vi "App - analyze RUS V6.vi"() -> ()   [LabVIEW 2015] (continued)
130814c\\5_Cooling_2nd_try\\September_2014\\091814\\14.36300K_500_2500_2.10000V_0.00000T_Sep18-2014__03-39-41_001_091814.bin", "mod time(min)"=58231179.68333333, "file format"=enum."binary", "power(V)"=2.1, "Magn Field(T) "=0.0}, {"temperature"=14.363, "temperature str"="14.36300", "file path"=path "D:/Data/Ultrasound/LSCO/LSCO22__130814c/5_Cooling_2nd_try/September_2014/091814/14.36300K_500_2500_2.10000V_0.00000T_Sep18-2014__03-41-00_001_091814.bin", "last mod"=timestamp(3493870860 s since 1904-01-01), "file name str"="D:\\Data\\Ultrasound\\LSCO\\LSCO22__130814c\\5_Cooling_2nd_try\\September_2014\\091814\\14.36300K_500_2500_2.10000V_0.00000T_Sep18-2014__03-41-00_001_091814.bin", "mod time(min)"=58231181.0, "file format"=enum."binary", "power(V)"=2.1, "Magn Field(T) "=0.0}, {"temperature"=14.36, "temperature str"="14.36000", "file path"=path "D:/Data/Ultrasound/LSCO/LSCO22__130814c/5_Cooling_2nd_try/September_2014/091814/14.36000K_500_2500_2.10000V_0.00000T_Sep18-2014__03-42-19_001_091814.bin", "last mod"=timestamp(3493870939 s since 1904-01-01), "file name str"="D:\\Data\\Ultrasound\\LSCO\\LSCO22__130814c\\5_Cooling_2nd_try\\September_2014\\091814\\14.36000K_500_2500_2.10000V_0.00000T_Sep18-2014__03-42-19_001_091814.bin", "mod time(min)"=58231182.31666667, "file format"=enum."binary", "power(V)"=2.1, "Magn Field(T) "=0.0}, {"temperature"=14.361, "temperature str"="14.36100", "file path"=path "D:/Data/Ultrasound/LSCO/LSCO22__130814c/5_Cooling_2nd_try/September_2014/091814/14.36100K_500_2500_2.10000V_0.00000T_Sep18-2014__03-43-39_001_091814.bin", "last mod"=timestamp(3493871019 s since 1904-01-01), "file name str"="D:\\Data\\Ultrasound\\LSCO\\LSCO22__130814c\\5_Cooling_2nd_try\\September_2014\\091814\\14.36100K_500_2500_2.10000V_0.00000T_Sep18-2014__03-43-39_001_091814.bin", "mod time(min)"=58231183.65, "file format"=enum."binary", "power(V)"=2.1, "Magn Field(T) "=0.0}, {"temperature"=14.361, "temperature str"="14.36100", "file path"=path "D:/Data/Ultrasound/LSCO/LSCO22__130814c/5_Cooling_2nd_try/September_2014/091814/14.36100K_500_2500_2.10000V_0.00000T_Sep18-2014__03-44-58_001_091814.bin", "last mod"=timestamp(3493871098 s since 1904-01-01), "file name str"="D:\\Data\\Ultrasound\\LSCO\\LSCO22__130814c\\5_Cooling_2nd_try\\September_2014\\091814\\14.36100K_500_2500_2.10000V_0.00000T_Sep18-2014__03-44-58_001_091814.bin", "mod time(min)"=58231184.96666667, "file format"=enum."binary", "power(V)"=2.1, "Magn Field(T) "=0.0}, {"temperature"=14.357, "temperature str"="14.35700", "file path"=path "D:/Data/Ultrasound/LSCO/LSCO22__130814c/5_Cooling_2nd_try/September_2014/091814/14.35700K_500_2500_2.10000V_0.00000T_Sep18-2014__03-46-18_001_091814.bin", "last mod"=timestamp(3493871178 s since 1904-01-01), "file name str"="D:\\Data\\Ultrasound\\LSCO\\LSCO22__130814c\\5_Cooling_2nd_try\\September_2014\\091814\\14.35700K_500_2500_2.10000V_0.00000T_Sep18-2014__03-46-18_001_091814.bin", "mod time(min)"=58231186.3, "file format"=enum."binary", "power(V)"=2.1, "Magn Field(T) "=0.0}, {"temperature"=14.357, "temperature str"="14.35700", "file path"=path "D:/Data/Ultrasound/LSCO/LSCO22__130814c/5_Cooling_2nd_try/September_2014/091814/14.35700K_500_2500_2.10000V_0.00000T_Sep18-2014__03-47-37_001_091814.bin", "last mod"=timestamp(3493871257 s since 1904-01-01), "file name str"="D:\\Data\\Ultrasound\\LSCO\\LSCO22__130814c\\5_Cooling_2nd_try\\September_2014\\091814\\14.35700K_500_2500_2.10000V_0.00000T_Sep18-2014__03-47-37_001_091814.bin", "mod time(min)"=58231187.61666667, "file format"=enum."binary", "power(V)"=2.1, "Magn Field(T) "=0.0}, {"temperature"=14.355, "temperature str"="14.35500", "file path"=path "D:/Data/Ultrasound/LSCO/LSCO22__130814c/5_Cooling_2nd_try/September_2014/091814/14.35500K_500_2500_2.10000V_0.00000T_Sep18-2014__03-48-56_001_091814.bin", "last mod"=timestamp(3493871336 s since 1904-01-01), "file name str"="D:\\Data\\Ultrasound\\LSCO\\LSCO22__130814c\\5_Cooling_2nd_try\\September_2014\\091814\\14.35500K_500_2500_2.10000V_0.00000T_Sep18-2014__03-48-56_001_091814.bin", "mod time(min)"=58231188.93333333, "file format"=enum."binary", "power(V)"=2.1, "Magn Field(T) "=0.0}, {"temperature"=14.354, "temperature str"="14.35400", "file path"=path "D:/Data/Ultrasound/LSCO/LSCO22__130814c/5_Cooling_2nd_try/September_2014/091814/14.35400K_500_2500_2.10000V_0.00000T_Sep18-2014__03-50-16_001_091814.bin", "last mod"=timestamp(3493871416 s since 1904-01-01), "file name str"="D:\\Data\\Ultrasound\\LSCO\\LSCO22__130814c\\5_Cooling_2nd_try\\September_2014\\091814\\14.35400K_500_2500_2.10000V_0.00000T_Sep18-2014__03-50-16_001_091814.bin", "mod time(min)"=58231190.266666666, "file format"=enum."binary", "power(V)"=2.1, "Magn Field(T) "=0.0}, {"temperature"=14.354, "temperature str"="14.35400", "file path"=path "D:/Data/Ultrasound/LSCO/LSCO22__130814c/5_Cooling_2nd_try/September_2014/091814/14.35400K_500_2500_2.10000V_0.00000T_Sep18-2014__03-51-35_001_091814.bin", "last mod"=timestamp(3493871495 s since 1904-01-01), "file name str"="D:\\Data\\Ultrasound\\LSCO\\LSCO22__130814c\\5_Cooling_2nd_try\\September_2014\\091814\\14.35400K_500_2500_2.10000V_0.00000T_Sep18-2014__03-51-35_001_091814.bin", "mod time(min)"=58231191.583333336, "file format"=enum."binary", "power(V)"=2.1, "Magn Field(T) "=0.0}, {"temperature"=14.352, "temperature str"="14.35200", "file path"=path "D:/Data/Ultrasound/LSCO/LSCO22__130814c/5_Cooling_2nd_try/September_2014/091814/14.35200K_500_2500_2.10000V_0.00000T_Sep18-2014__03-52-54_001_091814.bin", "last mod"=timestamp(3493871574 s since 1904-01-01), "file name str"="D:\\Data\\Ultrasound\\LSCO\\LSCO22__130814c\\5_Cooling_2nd_try\\September_2014\\091814\\14.35200K_500_2500_2.10000V_0.00000T_Sep18-2014__03-52-54_001_091814.bin", "mod time(min)"=58231192.9, "file format"=enum."binary", "power(V)"=2.1, "Magn Field(T) "=0.0}, {"temperature"=14.349, "temperature str"="14.34900", "file path"=path "D:/Data/Ultrasound/LSCO/LSCO22__130814c/5_Cooling_2nd_try/September_2014/091814/14.34900K_500_2500_2.10000V_0.00000T_Sep18-2014__03-54-14_001_091814.bin", "last mod"=timestamp(3493871654 s since 1904-01-01), "file name str"="D:\\Data\\Ultrasound\\LSCO\\LSCO22__130814c\\5_Cooling_2nd_try\\September_2014\\091814\\14.34900K_500_2500_2.10000V_0.00000T_Sep18-2014__03-54-14_001_091814.bin", "mod time(min)"=58231194.233333334, "file format"=enum."binary", "power(V)"=2.1, "Magn Field(T) "=0.0}, {"temperature"=14.353, "temperature str"="14.35300", "file path"=path "D:/Data/Ultrasound/LSCO/LSCO22__130814c/5_Cooling_2nd_try/September_2014/091814/14.35300K_500_2500_2.10000V_0.00000T_Sep18-2014__03-55-33_001_091814.bin", "last mod"=timestamp(3493871733 s since 1904-01-01), "file name str"="D:\\Data\\Ultrasound\\LSCO\\LSCO22__130814c\\5_Cooling_2nd_try\\September_2014\\091814\\14.35300K_500_2500_2.10000V_0.00000T_Sep18-2014__03-55-33_001_091814.bin", "mod time(min)"=58231195.55, "file format"=enum."binary", "power(V)"=2.1, "Magn Field(T) "=0.0}, {"temperature"=14.35, "temperature str"="14.35000", "file path"=path "D:/Data/Ultrasound/LSCO/LSCO22__130814c/5_Cooling_2nd_try/September_2014/091814/14.35000K_500_2500_2.10000V_0.00000T_Sep18-2014__03-56-53_001_091814.bin", "last mod"=timestamp(3493871813 s since 1904-01-01), "file name str"="D:\\Data\\Ultrasound\\LSCO\\LSCO22__130814c\\5_Cooling_2nd_try\\September_2014\\091814\\14.35000K_500_2500_2.10000V_0.00000T_Sep18-2014__03-56-53_001_091814.bin", "mod time(min)"=58231196.88333333, "file format"=enum."binary", "power(V)"=2.1, "Magn Field(T) "=0.0}, {"temperature"=14.351, "temperature str"="14.35100", "file path"=path "D:/Data/Ultrasound/LSCO/LSCO22__130814c/5_Cooling_2nd_try/September_2014/091814/14.35100K_500_2500_2.10000V_0.00000T_Sep18-2014__03-58-12_001_091814.bin", "last mod"=timestamp(3493871892 s since 1904-01-01), "file name str"="D:\\Data\\Ultrasound\\LSCO\\LSCO22__130814c\\5_Cooling_2nd_try\\September_2014\\091814\\14.35100K_500_2500_2.10000V_0.00000T_Sep18-2014__03-58-12_001_091814.bin", "mod time(min)"=58231198.2, "file format"=enum."binary", "power(V)"=2.1, "Magn Field(T) "=0.0}, {"temperature"=14.351, "temperature str"="14.35100", "file path"=path "D:/Data/Ultrasound/LSCO/LSCO22__130814c/5_Cooling_2nd_try/September_2014/091814/14.35100K_500_2500_2.10000V_0.00000T_Sep18-2014__03-59-31_001_091814.bin", "last mod"=timestamp(3493871971 s since 1904-01-01), "file name str"="D:\\Data\\Ultrasound\\LSCO\\LSCO22__130814c\\5_Cooling_2nd_try\\September_2014\\091814\\14.35100K_500_2500_2.10000V_0.00000T_Sep18-2014__03-59-31_001_091814.bin", "mod time(min)"=58231199.516666666, "file format"=enum."binary", "power(V)"=2.1, "Magn Field(T) "=0.0}, {"temperature"=14.353, "temperature str"="14.35300", "file path"=path "D:/Data/Ultrasound/LSCO/LSCO22__130814c/5_Cooling_2nd_try/September_2014/091814/14.35300K_500_2500_2.10000V_0.00000T_Sep18-2014__04-00-51_001_091814.bin", "last mod"=timestamp(3493872051 s since 1904-01-01), "file name str"="D:\\Data\\Ultrasound\\LSCO\\LSCO22__130814c\\5_Cooling_2nd_try\\September_2014\\091814\\14.35300K_500_2500_2.10000V_0.00000T_Sep18-2014__04-00-51_001_091814.bin", "mod time(min)"=58231200.85, "file format"=enum."binary", "power(V)"=2.1, "Magn Field(T) "=0.0}, {"temperature"=14.352, "temperature str"="14.35200", "file path"=path "D:/Data/Ultrasound/LSCO/LSCO22__130814c/5_Cooling_2nd_try/September_2014/091814/14.35200K_500_2500_2.10000V_0.00000T_Sep18-2014__04-02-10_001_091814.bin", "last mod"=timestamp(3493872130 s since 1904-01-01), "file name str"="D:\\Data\\Ultrasound\\LSCO\\LSCO22__130814c\\5_Cooling_2nd_try\\September_2014\\091814\\14.35200K_500_2500_2.10000V_0.00000T_Sep18-2014__04-02-10_001_091814.bin", "mod time(min)"=58231202.166666664, "file format"=enum."binary", "power(V)"=2.1, "Magn Field(T) "=0.0}, {"temperature"=14.354, "temperature str"="14.35400", "file path"=path "D:/Data/Ultrasound/LSCO/LSCO22__130814c/5_Cooling_2nd_try/September_2014/091814/14.35400K_500_2500_2.10000V_0.00000T_Sep18-2014__04-03-30_001_091814.bin", "last mod"=timestamp(3493872210 s since 1904-01-01), "file name str"="D:\\Data\\Ultrasound\\LSCO\\LSCO22__130814c\\5_Cooling_2nd_try\\September_2014\\091814\\14.35400K_500_2500_2.10000V_0.00000T_Sep18-2014__04-03-30_001_091814.bin", "mod time(min)"=58231203.5, "file format"=enum."binary", "power(V)"=2.1, "Magn Field(T) "=0.0}, {"temperature"=14.354, "temperature str"="14.35400", "file path"=path "D:/Data/Ultrasound/LSCO/LSCO22__130814c/5_Cooling_2nd_try/September_2014/091814/14.35400K_500_2500_2.10000V_0.00000T_Sep18-2014__04-04-49_001_091814.bin", "last mod"=timestamp(3493872289 s since 1904-01-01), "file name str"="D:\\Data\\Ultrasound\\LSCO\\LSCO22__130814c\\5_Cooling_2nd_try\\September_2014\\091814\\14.35400K_500_2500_2.10000V_0.00000T_Sep18-2014__04-04-49_001_091814.bin", "mod time(min)"=58231204.81666667, "file format"=enum."binary", "power(V)"=2.1, "Magn Field(T) "=0.0}, {"temperature"=14.358, "temperature str"="14.35800", "file path"=path "D:/Data/Ultrasound/LSCO/LSCO22__130814c/5_Cooling_2nd_try/September_2014/091814/14.35800K_500_2500_2.10000V_0.00000T_Sep18-2014__04-06-08_001_091814.bin", "last mod"=timestamp(3493872368 s since 1904-01-01), "file name str"="D:\\Data\\Ultrasound\\LSCO\\LSCO22__130814c\\5_Cooling_2nd_try\\September_2014\\091814\\14.35800K_500_2500_2.10000V_0.00000T_Sep18-2014__04-06-08_001_091814.bin", "mod time(min)"=58231206.13333333, "file format"=enum."binary", "power(V)"=2.1, "Magn Field(T) "=0.0}, {"temperature"=14.357, "temperature str"="14.35700", "file path"=path "D:/Data/Ultrasound/LSCO/LSCO22__130814c/5_Cooling_2nd_try/September_2014/091814/14.35700K_500_2500_2.10000V_0.00000T_Sep18-2014__04-07-28_001_091814.bin", "last mod"=timestamp(3493872448 s since 1904-01-01), "file name str"="D:\\Data\\Ultrasound\\LSCO\\LSCO22__130814c\\5_Cooling_2nd_try\\September_2014\\091814\\14.35700K_500_2500_2.10000V_0.00000T_Sep18-2014__04-07-28_001_091814.bin", "mod time(min)"=58231207.46666667, "file format"=enum."binary", "power(V)"=2.1, "Magn Field(T) "=0.0}, {"temperature"=14.356, "temperature str"="14.35600", "file path"=path "D:/Data/Ultrasound/LSCO/LSCO22__130814c/5_Cooling_2nd_try/September_2014/091814/14.35600K_500_2500_2.10000V_0.00000T_Sep18-2014__04-08-47_001_091814.bin", "last mod"=timestamp(3493872527 s since 1904-01-01), "file name str"="D:\\Data\\Ultrasound\\LSCO\\LSCO22__130814c\\5_Cooling_2nd_try\\September_2014\\091814\\14.35600K_500_2500_2.10000V_0.00000T_Sep18-2014__04-08-47_001_091814.bin", "mod time(min)"=58231208.78333333, "file format"=enum."binary", "power(V)"=2.1, "Magn Field(T) "=0.0}, {"temperature"=14.356, "temperature str"="14.35600", "file path"=path "D:/Data/Ultrasound/LSCO/LSCO22__130814c/5_Cooling_2nd_try/September_2014/091814/14.35600K_500_2500_2.10000V_0.00000T_Sep18-2014__04-10-06_001_091814.bin", "last mod"=timestamp(3493872606 s since 1904-01-01), "file name str"="D:\\Data\\Ultrasound\\LSCO\\LSCO22__130814c\\5_Cooling_2nd_try\\September_2014\\091814\\14.35600K_500_2500_2.10000V_0.00000T_Sep18-2014__04-10-06_001_091814.bin", "mod time(min)"=58231210.1, "file format"=enum."binary", "power(V)"=2.1, "Magn Field(T) "=0.0}, {"temperature"=14.354, "temperature str"="14.35400", "file path"=path "D:/Data/Ultrasound/LSCO/LSCO22__130814c/5_Cooling_2nd_try/September_2014/091814/14.35400K_500_2500_2.10000V_0.00000T_Sep18-2014__04-11-26_001_091814.bin", "last mod"=timestamp(3493872686 s since 1904-01-01), "file name str"="D:\\Data\\Ultrasound\\LSCO\\LSCO22__130814c\\5_Cooling_2nd_try\\September_2014\\091814\\14.35400K_500_2500_2.10000V_0.00000T_Sep18-2014__04-11-26_001_091814.bin", "mod time(min)"=58231211.43333333, "file format"=enum."binary", "power(V)"=2.1, "Magn Field(T) "=0.0}, {"temperature"=14.35, "temperature str"="14.35000", "file path"=path "D:/Data/Ultrasound/LSCO/LSCO22__130814c/5_Cooling_2nd_try/September_2014/091814/14.35000K_500_2500_2.10000V_0.00000T_Sep18-2014__04-12-45_001_091814.bin", "last mod"=timestamp(3493872765 s since 1904-01-01), "file name str"="D:\\Data\\Ultrasound\\LSCO\\LSCO22__130814c\\5_Cooling_2nd_try\\September_2014\\091814\\14.35000K_500_2500_2.10000V_0.00000T_Sep18-2014__04-12-45_001_091814.bin", "mod time(min)"=58231212.75, "file format"=enum."binary", "power(V)"=2.1, "Magn Field(T) "=0.0}, {"temperature"=14.352, "temperature str"="14.35200", "file path"=path "D:/Data/Ultrasound/LSCO/LSCO22__130814c/5_Cooling_2nd_try/September_2014/091814/14.35200K_500_2500_2.10000V_0.00000T_Sep18-2014__04-14-05_001_091814.bin", "last mod"=timestamp(3493872845 s since 1904-01-01), "file name str"="D:\\Data\\Ultrasound\\LSCO\\LSCO22__130814c\\5_Cooling_2nd_try\\September_2014\\091814\\14.35200K_500_2500_2.10000V_0.00000T_Sep18-2014__04-14-05_001_091814.bin", "mod time(min)"=58231214.083333336, "file format"=enum."binary", "power(V)"=2.1, "Magn Field(T) "=0.0}, {"temperature"=14.354, "temperature str"="14.35400", "file path"=path "D:/Data/Ultrasound/LSCO/LSCO22__130814c/5_Cooling_2nd_try/September_2014/091814/14.35400K_500_2500_2.10000V_0.00000T_Sep18-2014__04-15-24_001_091814.bin", "last mod"=timestamp(3493872924 s since 1904-01-01), "file name str"="D:\\Data\\Ultrasound\\LSCO\\LSCO22__130814c\\5_Cooling_2nd_try\\September_2014\\091814\\14.35400K_500_2500_2.10000V_0.00000T_Sep18-2014__04-15-24_001_091814.bin", "mod time(min)"=58231215.4, "file format"=enum."binary", "power(V)"=2.1, "Magn Field(T) "=0.0}, {"temperature"=14.349, "temperature str"="14.34900", "file path"=path "D:/Data/Ultrasound/LSCO/LSCO22__130814c/5_Cooling_2nd_try/September_2014/091814/14.34900K_500_2500_2.10000V_0.00000T_Sep18-2014__04-16-43_001_091814.bin", "last mod"=timestamp(3493873003 s since 1904-01-01), "file name str"="D:\\Data\\Ultrasound\\LSCO\\LSCO22__130814c\\5_Cooling_2nd_try\\September_2014\\091814\\14.34900K_500_2500_2.10000V_0.00000T_Sep18-2014__04-16-43_001_091814.bin", "mod time(min)"=58231216.71666667, "file format"=enum."binary", "power(V)"=2.1, "Magn Field(T) "=0.0}, {"temperature"=14.349, "temperature str"="14.34900", "file path"=path "D:/Data/Ultrasound/LSCO/LSCO22__130814c/5_Cooling_2nd_try/September_2014/091814/14.34900K_500_2500_2.10000V_0.00000T_Sep18-2014__04-18-03_001_091814.bin", "last mod"=timestamp(3493873083 s since 1904-01-01), "file name str"="D:\\Data\\Ultrasound\\LSCO\\LSCO22__130814c\\5_Cooling_2nd_try\\September_2014\\091814\\14.34900K_500_2500_2.10000V_0.00000T_Sep18-2014__04-18-03_001_091814.bin", "mod time(min)"=58231218.05, "file format"=enum."binary", "power(V)"=2.1, "Magn Field(T) "=0.0}, {"temperature"=14.346, "temperature str"="14.34600", "file path"=path "D:/Data/Ultrasound/LSCO/LSCO22__130814c/5_Cooling_2nd_try/September_2014/091814/14.34600K_500_2500_2.10000V_0.00000T_Sep18-2014__04-19-22_001_091814.bin", "last mod"=timestamp(3493873162 s since 1904-01-01), "file name str"="D:\\Data\\Ultrasound\\LSCO\\LSCO22__130814c\\5_Cooling_2nd_try\\September_2014\\091814\\14.34600K_500_2500_2.10000V_0.00000T_Sep18-2014__04-19-22_001_091814.bin", "mod time(min)"=58231219.36666667, "file format"=enum."binary", "power(V)"=2.1, "Magn Field(T) "=0.0}, {"temperature"=14.344, "temperature str"="14.34400", "file path"=path "D:/Data/Ultrasound/LSCO/LSCO22__130814c/5_Cooling_2nd_try/September_2014/091814/14.34400K_500_2500_2.10000V_0.00000T_Sep18-2014__04-20-42_001_091814.bin", "last mod"=timestamp(3493873242 s since 1904-01-01), "file name str"="D:\\Data\\Ultrasound\\LSCO\\LSCO22__130814c\\5_Cooling_2nd_try\\September_2014\\091814\\14.34400K_500_2500_2.10000V_0.00000T_Sep18-2014__04-20-42_001_091814.bin", "mod time(min)"=58231220.7, "file format"=enum."binary", "power(V)"=2.1, "Magn Field(T) "=0.0}, {"temperature"=14.346, "temperature str"="14.34600", "file path"=path "D:/Data/Ultrasound/LSCO/LSCO22__130814c/5_Cooling_2nd_try/September_2014/091814/14.34600K_500_2500_2.10000V_0.00000T_Sep18-2014__04-22-01_001_091814.bin", "last mod"=timestamp(3493873321 s since 1904-01-01), "file name str"="D:\\Data\\Ultrasound\\LSCO\\LSCO22__130814c\\5_Cooling_2nd_try\\September_2014\\091814\\14.34600K_500_2500_2.10000V_0.00000T_Sep18-2014__04-22-01_001_091814.bin", "mod time(min)"=58231222.016666666, "file format"=enum."binary", "power(V)"=2.1, "Magn Field(T) "=0.0}, {"temperature"=14.346, "temperature str"="14.34600", "file path"=path "D:/Data/Ultrasound/LSCO/LSCO22__130814c/5_Cooling_2nd_try/September_2014/091814/14.34600K_500_2500_2.10000V_0.00000T_Sep18-2014__04-23-20_001_091814.bin", "last mod"=timestamp(3493873400 s since 1904-01-01), "file name str"="D:\\Data\\Ultrasound\\LSCO\\LSCO22__130814c\\5_Cooling_2nd_try\\September_2014\\091814\\14.34600K_500_2500_2.10000V_0.00000T_Sep18-2014__04-23-20_001_091814.bin", "mod time(min)"=58231223.333333336, "file format"=enum."binary", "power(V)"=2.1, "Magn Field(T) "=0.0}, {"temperature"=14.348, "temperature str"="14.34800", "file path"=path "D:/Data/Ultrasound/LSCO/LSCO22__130814c/5_Cooling_2nd_try/September_2014/091814/14.34800K_500_2500_2.10000V_0.00000T_Sep18-2014__04-24-40_001_091814.bin", "last mod"=timestamp(3493873480 s since 1904-01-01), "file name str"="D:\\Data\\Ultrasound\\LSCO\\LSCO22__130814c\\5_Cooling_2nd_try\\September_2014\\091814\\14.34800K_500_2500_2.10000V_0.00000T_Sep18-2014__04-24-40_001_091814.bin", "mod time(min)"=58231224.666666664, "file format"=enum."binary", "power(V)"=2.1, "Magn Field(T) "=0.0}, {"temperature"=14.353, "temperature str"="14.35300", "file path"=path "D:/Data/Ultrasound/LSCO/LSCO22__130814c/5_Cooling_2nd_try/September_2014/091814/14.35300K_500_2500_2.10000V_0.00000T_Sep18-2014__04-25-59_001_091814.bin", "last mod"=timestamp(3493873559 s since 1904-01-01), "file name str"="D:\\Data\\Ultrasound\\LSCO\\LSCO22__130814c\\5_Cooling_2nd_try\\September_2014\\091814\\14.35300K_500_2500_2.10000V_0.00000T_Sep18-2014__04-25-59_001_091814.bin", "mod time(min)"=58231225.983333334, "file format"=enum."binary", "power(V)"=2.1, "Magn Field(T) "=0.0}, {"temperature"=14.355, "temperature str"="14.35500", "file path"=path "D:/Data/Ultrasound/LSCO/LSCO22__130814c/5_Cooling_2nd_try/September_2014/091814/14.35500K_500_2500_2.10000V_0.00000T_Sep18-2014__04-27-18_001_091814.bin", "last mod"=timestamp(3493873638 s since 1904-01-01), "file name str"="D:\\Data\\Ultrasound\\LSCO\\LSCO22__130814c\\5_Cooling_2nd_try\\September_2014\\091814\\14.35500K_500_2500_2.10000V_0.00000T_Sep18-2014__04-27-18_001_091814.bin", "mod time(min)"=58231227.3, "file format"=enum."binary", "power(V)"=2.1, "Magn Field(T) "=0.0}, {"temperature"=14.349, "temperature str"="14.34900", "file path"=path "D:/Data/Ultrasound/LSCO/LSCO22__130814c/5_Cooling_2nd_try/September_2014/091814/14.34900K_500_2500_2.10000V_0.00000T_Sep18-2014__04-28-38_001_091814.bin", "last mod"=timestamp(3493873718 s since 1904-01-01), "file name str"="D:\\Data\\Ultrasound\\LSCO\\LSCO22__130814c\\5_Cooling_2nd_try\\September_2014\\091814\\14.34900K_500_2500_2.10000V_0.00000T_Sep18-2014__04-28-38_001_091814.bin", "mod time(min)"=58231228.63333333, "file format"=enum."binary", "power(V)"=2.1, "Magn Field(T) "=0.0}, {"temperature"=14.351, "temperature str"="14.35100", "file path"=path "D:/Data/Ultrasound/LSCO/LSCO22__130814c/5_Cooling_2nd_try/September_2014/091814/14.35100K_500_2500_2.10000V_0.00000T_Sep18-2014__04-29-57_001_091814.bin", "last mod"=timestamp(3493873797 s since 1904-01-01), "file name str"="D:\\Data\\Ultrasound\\LSCO\\LSCO22__130814c\\5_Cooling_2nd_try\\September_2014\\091814\\14.35100K_500_2500_2.10000V_0.00000T_Sep18-2014__04-29-57_001_091814.bin", "mod time(min)"=58231229.95, "file format"=enum."binary", "power(V)"=2.1, "Magn Field(T) "=0.0}, {"temperature"=14.35, "temperature str"="14.35000", "file path"=path "D:/Data/Ultrasound/LSCO/LSCO22__130814c/5_Cooling_2nd_try/September_2014/091814/14.35000K_500_2500_2.10000V_0.00000T_Sep18-2014__04-31-17_001_091814.bin", "last mod"=timestamp(3493873877 s since 1904-01-01), "file name str"="D:\\Data\\Ultrasound\\LSCO\\LSCO22__130814c\\5_Cooling_2nd_try\\September_2014\\091814\\14.35000K_500_2500_2.10000V_0.00000T_Sep18-2014__04-31-17_001_091814.bin", "mod time(min)"=58231231.28333333, "file format"=enum."binary", "power(V)"=2.1, "Magn Field(T) "=0.0}, {"temperature"=14.347, "temperature str"="14.34700", "file path"=path "D:/Data/Ultrasound/LSCO/LSCO22__130814c/5_Cooling_2nd_try/September_2014/091814/14.34700K_500_2500_2.10000V_0.00000T_Sep18-2014__04-32-36_001_091814.bin", "last mod"=timestamp(3493873956 s since 1904-01-01), "file name str"="D:\\Data\\Ultrasound\\LSCO\\LSCO22__130814c\\5_Cooling_2nd_try\\September_2014\\091814\\14.34700K_500_2500_2.10000V_0.00000T_Sep18-2014__04-32-36_001_091814.bin", "mod time(min)"=58231232.6, "file format"=enum."binary", "power(V)"=2.1, "Magn Field(T) "=0.0}, {"temperature"=14.35, "temperature str"="14.35000", "file path"=path "D:/Data/Ultrasound/LSCO/LSCO22__130814c/5_Cooling_2nd_try/September_2014/091814/14.35000K_500_2500_2.10000V_0.00000T_Sep18-2014__04-33-55_001_091814.bin", "last mod"=timestamp(3493874035 s since 1904-01-01), "file name str"="D:\\Data\\Ultrasound\\LSCO\\LSCO22__130814c\\5_Cooling_2nd_try\\September_2014\\091814\\14.35000K_500_2500_2.10000V_0.00000T_Sep18-2014__04-33-55_001_091814.bin", "mod time(min)"=58231233.916666664, "file format"=enum."binary", "power(V)"=2.1, "Magn Field(T) "=0.0}, {"temperature"=14.349, "temperature str"="14.34900", "file path"=path "D:/Data/Ultrasound/LSCO/LSCO22__130814c/5_Cooling_2nd_try/September_2014/091814/14.34900K_500_2500_2.10000V_0.00000T_Sep18-2014__04-35-15_001_091814.bin", "last mod"=timestamp(3493874115 s since 1904-01-01), "file name str"="D:\\Data\\Ultrasound\\LSCO\\LSCO22__130814c\\5_Cooling_2nd_try\\September_2014\\091814\\14.34900K_500_2500_2.10000V_0.00000T_Sep18-2014__04-35-15_001_091814.bin", "mod time(min)"=58231235.25, "file format"=enum."binary", "power(V)"=2.1, "Magn Field(T) "=0.0}, {"temperature"=14.35, "temperature str"="14.35000", "file path"=path "D:/Data/Ultrasound/LSCO/LSCO22__130814c/5_Cooling_2nd_try/September_2014/091814/14.35000K_500_2500_2.10000V_0.00000T_Sep18-2014__04-36-34_001_091814.bin", "last mod"=timestamp(3493874194 s since 1904-01-01), "file name str"="D:\\Data\\Ultrasound\\LSCO\\LSCO22__130814c\\5_Cooling_2nd_try\\September_2014\\091814\\14.35000K_500_2500_2.10000V_0.00000T_Sep18-2014__04-36-34_001_091814.bin", "mod time(min)"=58231236.56666667, "file format"=enum."binary", "power(V)"=2.1, "Magn Field(T) "=0.0}, {"temperature"=14.351, "temperature str"="14.35100", "file path"=path "D:/Data/Ultrasound/LSCO/LSCO22__130814c/5_Cooling_2nd_try/September_2014/091814/14.35100K_500_2500_2.10000V_0.00000T_Sep18-2014__04-37-53_001_091814.bin", "last mod"=timestamp(3493874273 s since 1904-01-01), "file name str"="D:\\Data\\Ultrasound\\LSCO\\LSCO22__130814c\\5_Cooling_2nd_try\\September_2014\\091814\\14.35100K_500_2500_2.10000V_0.00000T_Sep18-2014__04-37-53_001_091814.bin", "mod time(min)"=58231237.88333333, "file format"=enum."binary", "power(V)"=2.1, "Magn Field(T) "=0.0}, {"temperature"=14.351, "temperature str"="14.35100", "file path"=path "D:/Data/Ultrasound/LSCO/LSCO22__130814c/5_Cooling_2nd_try/September_2014/091814/14.35100K_500_2500_2.10000V_0.00000T_Sep18-2014__04-39-13_001_091814.bin", "last mod"=timestamp(3493874353 s since 1904-01-01), "file name str"="D:\\Data\\Ultrasound\\LSCO\\LSCO22__130814c\\5_Cooling_2nd_try\\September_2014\\091814\\14.35100K_500_2500_2.10000V_0.00000T_Sep18-2014__04-39-13_001_091814.bin", "mod time(min)"=58231239.21666667, "file format"=enum."binary", "power(V)"=2.1, "Magn Field(T) "=0.0}, {"temperature"=14.352, "temperature str"="14.35200", "file path"=path "D:/Data/Ultrasound/LSCO/LSCO22__130814c/5_Cooling_2nd_try/September_2014/091814/14.35200K_500_2500_2.10000V_0.00000T_Sep18-2014__04-40-32_001_091814.bin", "last mod"=timestamp(3493874432 s since 1904-01-01), "file name str"="D:\\Data\\Ultrasound\\LSCO\\LSCO22__130814c\\5_Cooling_2nd_try\\September_2014\\091814\\14.35200K_500_2500_2.10000V_0.00000T_Sep18-2014__04-40-32_001_091814.bin", "mod time(min)"=58231240.53333333, "file format"=enum."binary", "power(V)"=2.1, "Magn Field(T) "=0.0}, {"temperature"=14.351, "temperature str"="14.35100", "file path"=path "D:/Data/Ultrasound/LSCO/LSCO22__130814c/5_Cooling_2nd_try/September_2014/091814/14.35100K_500_2500_2.10000V_0.00000T_Sep18-2014__04-41-52_001_091814.bin", "last mod"=timestamp(3493874512 s since 1904-01-01), "file name str"="D:\\Data\\Ultrasound\\LSCO\\LSCO22__130814c\\5_Cooling_2nd_try\\September_2014\\091814\\14.35100K_500_2500_2.10000V_0.00000T_Sep18-2014__04-41-52_001_091814.bin", "mod time(min)"=58231241.86666667, "file format"=enum."binary", "power(V)"=2.1, "Magn Field(T) "=0.0}, {"temperature"=14.35, "temperature str"="14.35000", "file path"=path "D:/Data/Ultrasound/LSCO/LSCO22__130814c/5_Cooling_2nd_try/September_2014/091814/14.35000K_500_2500_2.10000V_0.00000T_Sep18-2014__04-43-11_001_091814.bin", "last mod"=timestamp(3493874591 s since 1904-01-01), "file name str"="D:\\Data\\Ultrasound\\LSCO\\LSCO22__130814c\\5_Cooling_2nd_try\\September_2014\\091814\\14.35000K_500_2500_2.10000V_0.00000T_Sep18-2014__04-43-11_001_091814.bin", "mod time(min)"=58231243.18333333, "file format"=enum."binary", "power(V)"=2.1, "Magn Field(T) "=0.0}, {"temperature"=14.353, "temperature str"="14.35300", "file path"=path "D:/Data/Ultrasound/LSCO/LSCO22__130814c/5_Cooling_2nd_try/September_2014/091814/14.35300K_500_2500_2.10000V_0.00000T_Sep18-2014__04-44-30_001_091814.bin", "last mod"=timestamp(3493874670 s since 1904-01-01), "file name str"="D:\\Data\\Ultrasound\\LSCO\\LSCO22__130814c\\5_Cooling_2nd_try\\September_2014\\091814\\14.35300K_500_2500_2.10000V_0.00000T_Sep18-2014__04-44-30_001_091814.bin", "mod time(min)"=58231244.5, "file format"=enum."binary", "power(V)"=2.1, "Magn Field(T) "=0.0}, {"temperature"=14.354, "temperature str"="14.35400", "file path"=path "D:/Data/Ultrasound/LSCO/LSCO22__130814c/5_Cooling_2nd_try/September_2014/091814/14.35400K_500_2500_2.10000V_0.00000T_Sep18-2014__04-45-50_001_091814.bin", "last mod"=timestamp(3493874750 s since 1904-01-01), "file name str"="D:\\Data\\Ultrasound\\LSCO\\LSCO22__130814c\\5_Cooling_2nd_try\\September_2014\\091814\\14.35400K_500_2500_2.10000V_0.00000T_Sep18-2014__04-45-50_001_091814.bin", "mod time(min)"=58231245.833333336, "file format"=enum."binary", "power(V)"=2.1, "Magn Field(T) "=0.0}, {"temperature"=14.356, "temperature str"="14.35600", "file path"=path "D:/Data/Ultrasound/LSCO/LSCO22__130814c/5_Cooling_2nd_try/September_2014/091814/14.35600K_500_2500_2.10000V_0.00000T_Sep18-2014__04-47-09_001_091814.bin", "last mod"=timestamp(3493874829 s since 1904-01-01), "file name str"="D:\\Data\\Ultrasound\\LSCO\\LSCO22__130814c\\5_Cooling_2nd_try\\September_2014\\091814\\14.35600K_500_2500_2.10000V_0.00000T_Sep18-2014__04-47-09_001_091814.bin", "mod time(min)"=58231247.15, "file format"=enum."binary", "power(V)"=2.1, "Magn Field(T) "=0.0}, {"temperature"=14.359, "temperature str"="14.35900", "file path"=path "D:/Data/Ultrasound/LSCO/LSCO22__130814c/5_Cooling_2nd_try/September_2014/091814/14.35900K_500_2500_2.10000V_0.00000T_Sep18-2014__04-48-29_001_091814.bin", "last mod"=timestamp(3493874909 s since 1904-01-01), "file name str"="D:\\Data\\Ultrasound\\LSCO\\LSCO22__130814c\\5_Cooling_2nd_try\\September_2014\\091814\\14.35900K_500_2500_2.10000V_0.00000T_Sep18-2014__04-48-29_001_091814.bin", "mod time(min)"=58231248.483333334, "file format"=enum."binary", "power(V)"=2.1, "Magn Field(T) "=0.0}, {"temperature"=14.361, "temperature str"="14.36100", "file path"=path "D:/Data/Ultrasound/LSCO/LSCO22__130814c/5_Cooling_2nd_try/September_2014/091814/14.36100K_500_2500_2.10000V_0.00000T_Sep18-2014__04-49-48_001_091814.bin", "last mod"=timestamp(3493874988 s since 1904-01-01), "file name str"="D:\\Data\\Ultrasound\\LSCO\\LSCO22__130814c\\5_Cooling_2nd_try\\September_2014\\091814\\14.36100K_500_2500_2.10000V_0.00000T_Sep18-2014__04-49-48_001_091814.bin", "mod time(min)"=58231249.8, "file format"=enum."binary", "power(V)"=2.1, "Magn Field(T) "=0.0}, {"temperature"=14.36, "temperature str"="14.36000", "file path"=path "D:/Data/Ultrasound/LSCO/LSCO22__130814c/5_Cooling_2nd_try/September_2014/091814/14.36000K_500_2500_2.10000V_0.00000T_Sep18-2014__04-51-07_001_091814.bin", "last mod"=timestamp(3493875067 s since 1904-01-01), "file name str"="D:\\Data\\Ultrasound\\LSCO\\LSCO22__130814c\\5_Cooling_2nd_try\\September_2014\\091814\\14.36000K_500_2500_2.10000V_0.00000T_Sep18-2014__04-51-07_001_091814.bin", "mod time(min)"=58231251.11666667, "file format"=enum."binary", "power(V)"=2.1, "Magn Field(T) "=0.0}, {"temperature"=14.364, "temperature str"="14.36400", "file path"=path "D:/Data/Ultrasound/LSCO/LSCO22__130814c/5_Cooling_2nd_try/September_2014/091814/14.36400K_500_2500_2.10000V_0.00000T_Sep18-2014__04-52-27_001_091814.bin", "last mod"=timestamp(3493875147 s since 1904-01-01), "file name str"="D:\\Data\\Ultrasound\\LSCO\\LSCO22__130814c\\5_Cooling_2nd_try\\September_2014\\091814\\14.36400K_500_2500_2.10000V_0.00000T_Sep18-2014__04-52-27_001_091814.bin", "mod time(min)"=58231252.45, "file format"=enum."binary", "power(V)"=2.1, "Magn Field(T) "=0.0}, {"temperature"=14.363, "temperature str"="14.36300", "file path"=path "D:/Data/Ultrasound/LSCO/LSCO22__130814c/5_Cooling_2nd_try/September_2014/091814/14.36300K_500_2500_2.10000V_0.00000T_Sep18-2014__04-53-46_001_091814.bin", "last mod"=timestamp(3493875226 s since 1904-01-01), "file name str"="D:\\Data\\Ultrasound\\LSCO\\LSCO22__130814c\\5_Cooling_2nd_try\\September_2014\\091814\\14.36300K_500_2500_2.10000V_0.00000T_Sep18-2014__04-53-46_001_091814.bin", "mod time(min)"=58231253.766666666, "file format"=enum."binary", "power(V)"=2.1, "Magn Field(T) "=0.0}, {"temperature"=14.368, "temperature str"="14.36800", "file path"=path "D:/Data/Ultrasound/LSCO/LSCO22__130814c/5_Cooling_2nd_try/September_2014/091814/14.36800K_500_2500_2.10000V_0.00000T_Sep18-2014__04-55-05_001_091814.bin", "last mod"=timestamp(3493875305 s since 1904-01-01), "file name str"="D:\\Data\\Ultrasound\\LSCO\\LSCO22__130814c\\5_Cooling_2nd_try\\September_2014\\091814\\14.36800K_500_2500_2.10000V_0.00000T_Sep18-2014__04-55-05_001_091814.bin", "mod time(min)"=58231255.083333336, "file format"=enum."binary", "power(V)"=2.1, "Magn Field(T) "=0.0}, {"temperature"=14.367, "temperature str"="14.36700", "file path"=path "D:/Data/Ultrasound/LSCO/LSCO22__130814c/5_Cooling_2nd_try/September_2014/091814/14.36700K_500_2500_2.10000V_0.00000T_Sep18-2014__04-56-25_001_091814.bin", "last mod"=timestamp(3493875385 s since 1904-01-01), "file name str"="D:\\Data\\Ultrasound\\LSCO\\LSCO22__130814c\\5_Cooling_2nd_try\\September_2014\\091814\\14.36700K_500_2500_2.10000V_0.00000T_Sep18-2014__04-56-25_001_091814.bin", "mod time(min)"=58231256.416666664, "file format"=enum."binary", "power(V)"=2.1, "Magn Field(T) "=0.0}, {"temperature"=14.368, "temperature str"="14.36800", "file path"=path "D:/Data/Ultrasound/LSCO/LSCO22__130814c/5_Cooling_2nd_try/September_2014/091814/14.36800K_500_2500_2.10000V_0.00000T_Sep18-2014__04-57-44_001_091814.bin", "last mod"=timestamp(3493875464 s since 1904-01-01), "file name str"="D:\\Data\\Ultrasound\\LSCO\\LSCO22__130814c\\5_Cooling_2nd_try\\September_2014\\091814\\14.36800K_500_2500_2.10000V_0.00000T_Sep18-2014__04-57-44_001_091814.bin", "mod time(min)"=58231257.733333334, "file format"=enum."binary", "power(V)"=2.1, "Magn Field(T) "=0.0}, {"temperature"=14.368, "temperature str"="14.36800", "file path"=path "D:/Data/Ultrasound/LSCO/LSCO22__130814c/5_Cooling_2nd_try/September_2014/091814/14.36800K_500_2500_2.10000V_0.00000T_Sep18-2014__04-59-04_001_091814.bin", "last mod"=timestamp(3493875544 s since 1904-01-01), "file name str"="D:\\Data\\Ultrasound\\LSCO\\LSCO22__130814c\\5_Cooling_2nd_try\\September_2014\\091814\\14.36800K_500_2500_2.10000V_0.00000T_Sep18-2014__04-59-04_001_091814.bin", "mod time(min)"=58231259.06666667, "file format"=enum."binary", "power(V)"=2.1, "Magn Field(T) "=0.0}, {"temperature"=14.366, "temperature str"="14.36600", "file path"=path "D:/Data/Ultrasound/LSCO/LSCO22__130814c/5_Cooling_2nd_try/September_2014/091814/14.36600K_500_2500_2.10000V_0.00000T_Sep18-2014__05-00-23_001_091814.bin", "last mod"=timestamp(3493875623 s since 1904-01-01), "file name str"="D:\\Data\\Ultrasound\\LSCO\\LSCO22__130814c\\5_Cooling_2nd_try\\September_2014\\091814\\14.36600K_500_2500_2.10000V_0.00000T_Sep18-2014__05-00-23_001_091814.bin", "mod time(min)"=58231260.38333333, "file format"=enum."binary", "power(V)"=2.1, "Magn Field(T) "=0.0}, {"temperature"=14.369, "temperature str"="14.36900", "file path"=path "D:/Data/Ultrasound/LSCO/LSCO22__130814c/5_Cooling_2nd_try/September_2014/091814/14.36900K_500_2500_2.10000V_0.00000T_Sep18-2014__05-01-42_001_091814.bin", "last mod"=timestamp(3493875702 s since 1904-01-01), "file name str"="D:\\Data\\Ultrasound\\LSCO\\LSCO22__130814c\\5_Cooling_2nd_try\\September_2014\\091814\\14.36900K_500_2500_2.10000V_0.00000T_Sep18-2014__05-01-42_001_091814.bin", "mod time(min)"=58231261.7, "file format"=enum."binary", "power(V)"=2.1, "Magn Field(T) "=0.0}, {"temperature"=14.369, "temperature str"="14.36900", "file path"=path "D:/Data/Ultrasound/LSCO/LSCO22__130814c/5_Cooling_2nd_try/September_2014/091814/14.36900K_500_2500_2.10000V_0.00000T_Sep18-2014__05-03-02_001_091814.bin", "last mod"=timestamp(3493875782 s since 1904-01-01), "file name str"="D:\\Data\\Ultrasound\\LSCO\\LSCO22__130814c\\5_Cooling_2nd_try\\September_2014\\091814\\14.36900K_500_2500_2.10000V_0.00000T_Sep18-2014__05-03-02_001_091814.bin", "mod time(min)"=58231263.03333333, "file format"=enum."binary", "power(V)"=2.1, "Magn Field(T) "=0.0}, {"temperature"=14.371, "temperature str"="14.37100", "file path"=path "D:/Data/Ultrasound/LSCO/LSCO22__130814c/5_Cooling_2nd_try/September_2014/091814/14.37100K_500_2500_2.10000V_0.00000T_Sep18-2014__05-04-21_001_091814.bin", "last mod"=timestamp(3493875861 s since 1904-01-01), "file name str"="D:\\Data\\Ultrasound\\LSCO\\LSCO22__130814c\\5_Cooling_2nd_try\\September_2014\\091814\\14.37100K_500_2500_2.10000V_0.00000T_Sep18-2014__05-04-21_001_091814.bin", "mod time(min)"=58231264.35, "file format"=enum."binary", "power(V)"=2.1, "Magn Field(T) "=0.0}, {"temperature"=14.377, "temperature str"="14.37700", "file path"=path "D:/Data/Ultrasound/LSCO/LSCO22__130814c/5_Cooling_2nd_try/September_2014/091814/14.37700K_500_2500_2.10000V_0.00000T_Sep18-2014__05-05-40_001_091814.bin", "last mod"=timestamp(3493875940 s since 1904-01-01), "file name str"="D:\\Data\\Ultrasound\\LSCO\\LSCO22__130814c\\5_Cooling_2nd_try\\September_2014\\091814\\14.37700K_500_2500_2.10000V_0.00000T_Sep18-2014__05-05-40_001_091814.bin", "mod time(min)"=58231265.666666664, "file format"=enum."binary", "power(V)"=2.1, "Magn Field(T) "=0.0}, {"temperature"=14.377, "temperature str"="14.37700", "file path"=path "D:/Data/Ultrasound/LSCO/LSCO22__130814c/5_Cooling_2nd_try/September_2014/091814/14.37700K_500_2500_2.10000V_0.00000T_Sep18-2014__05-07-00_001_091814.bin", "last mod"=timestamp(3493876020 s since 1904-01-01), "file name str"="D:\\Data\\Ultrasound\\LSCO\\LSCO22__130814c\\5_Cooling_2nd_try\\September_2014\\091814\\14.37700K_500_2500_2.10000V_0.00000T_Sep18-2014__05-07-00_001_091814.bin", "mod time(min)"=58231267.0, "file format"=enum."binary", "power(V)"=2.1, "Magn Field(T) "=0.0}, {"temperature"=14.374, "temperature str"="14.37400", "file path"=path "D:/Data/Ultrasound/LSCO/LSCO22__130814c/5_Cooling_2nd_try/September_2014/091814/14.37400K_500_2500_2.10000V_0.00000T_Sep18-2014__05-08-19_001_091814.bin", "last mod"=timestamp(3493876099 s since 1904-01-01), "file name str"="D:\\Data\\Ultrasound\\LSCO\\LSCO22__130814c\\5_Cooling_2nd_try\\September_2014\\091814\\14.37400K_500_2500_2.10000V_0.00000T_Sep18-2014__05-08-19_001_091814.bin", "mod time(min)"=58231268.31666667, "file format"=enum."binary", "power(V)"=2.1, "Magn Field(T) "=0.0}, {"temperature"=14.374, "temperature str"="14.37400", "file path"=path "D:/Data/Ultrasound/LSCO/LSCO22__130814c/5_Cooling_2nd_try/September_2014/091814/14.37400K_500_2500_2.10000V_0.00000T_Sep18-2014__05-09-39_001_091814.bin", "last mod"=timestamp(3493876179 s since 1904-01-01), "file name str"="D:\\Data\\Ultrasound\\LSCO\\LSCO22__130814c\\5_Cooling_2nd_try\\September_2014\\091814\\14.37400K_500_2500_2.10000V_0.00000T_Sep18-2014__05-09-39_001_091814.bin", "mod time(min)"=58231269.65, "file format"=enum."binary", "power(V)"=2.1, "Magn Field(T) "=0.0}, {"temperature"=14.376, "temperature str"="14.37600", "file path"=path "D:/Data/Ultrasound/LSCO/LSCO22__130814c/5_Cooling_2nd_try/September_2014/091814/14.37600K_500_2500_2.10000V_0.00000T_Sep18-2014__05-10-58_001_091814.bin", "last mod"=timestamp(3493876258 s since 1904-01-01), "file name str"="D:\\Data\\Ultrasound\\LSCO\\LSCO22__130814c\\5_Cooling_2nd_try\\September_2014\\091814\\14.37600K_500_2500_2.10000V_0.00000T_Sep18-2014__05-10-58_001_091814.bin", "mod time(min)"=58231270.96666667, "file format"=enum."binary", "power(V)"=2.1, "Magn Field(T) "=0.0}, {"temperature"=14.375, "temperature str"="14.37500", "file path"=path "D:/Data/Ultrasound/LSCO/LSCO22__130814c/5_Cooling_2nd_try/September_2014/091814/14.37500K_500_2500_2.10000V_0.00000T_Sep18-2014__05-12-17_001_091814.bin", "last mod"=timestamp(3493876337 s since 1904-01-01), "file name str"="D:\\Data\\Ultrasound\\LSCO\\LSCO22__130814c\\5_Cooling_2nd_try\\September_2014\\091814\\14.37500K_500_2500_2.10000V_0.00000T_Sep18-2014__05-12-17_001_091814.bin", "mod time(min)"=58231272.28333333, "file format"=enum."binary", "power(V)"=2.1, "Magn Field(T) "=0.0}, {"temperature"=14.379, "temperature str"="14.37900", "file path"=path "D:/Data/Ultrasound/LSCO/LSCO22__130814c/5_Cooling_2nd_try/September_2014/091814/14.37900K_500_2500_2.10000V_0.00000T_Sep18-2014__05-13-37_001_091814.bin", "last mod"=timestamp(3493876417 s since 1904-01-01), "file name str"="D:\\Data\\Ultrasound\\LSCO\\LSCO22__130814c\\5_Cooling_2nd_try\\September_2014\\091814\\14.37900K_500_2500_2.10000V_0.00000T_Sep18-2014__05-13-37_001_091814.bin", "mod time(min)"=58231273.61666667, "file format"=enum."binary", "power(V)"=2.1, "Magn Field(T) "=0.0}, {"temperature"=14.38, "temperature str"="14.38000", "file path"=path "D:/Data/Ultrasound/LSCO
